vi "Create Parser.vi"(8 "error in (no error)":errorcluster, 10 "LVLIBP Path":path) -> (0 "error out":errorcluster, 3 "LVLIBP Parser out":refnum<class "LVLIBP Parser.lvclass">)   [LabVIEW 2020, in "LVLIBP CD XML Updater.lvlib" / "LVLIBP Parser.lvclass"]
uses:
  LVLIBP Parser.lvclass
  LVLIBP Parser.lvclass/LVLIBP Parser.ctl
  <vilib>/Utility/LVLibp/NI_PackedLibraryUtility.lvlib
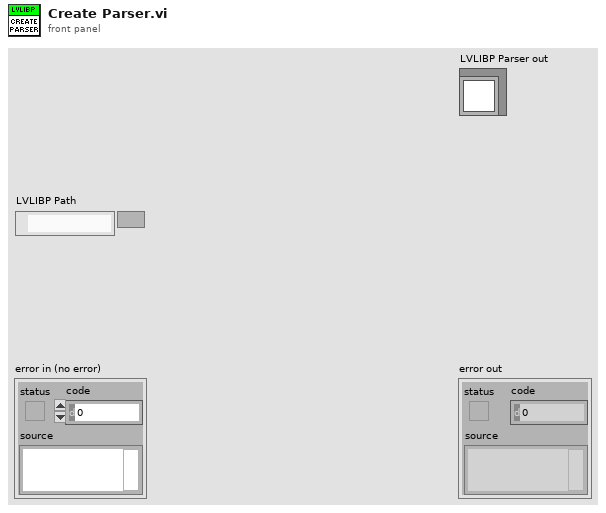
[diagram p1: front panel]
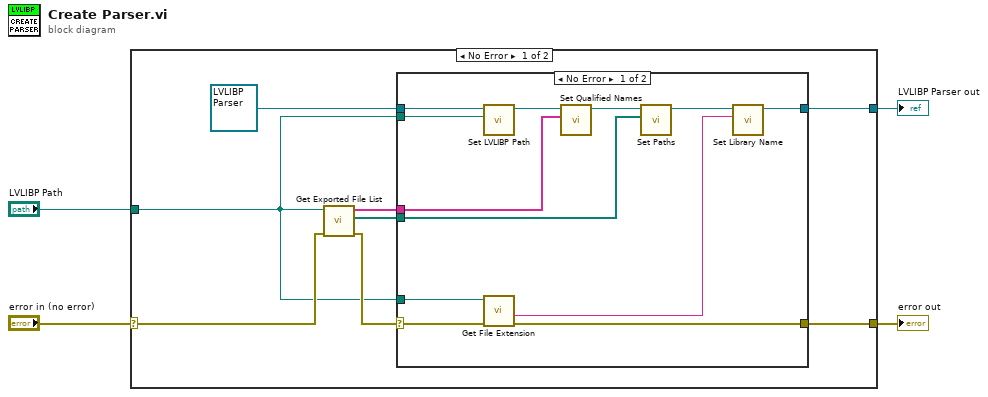
[diagram p0: block diagram]
diagram:
  n1 = case shown="No Error" "error in (no error)" {
    selector: "error in (no error)" -> [w10 w27]
    tunnel: [w8 w27] -> w3
    tunnel: "LVLIBP Path" -> [w5 _]
    tunnel: [w11 _] -> w1
    frame No Error {
      n2 = call <vilib>:"Get Exported File List.vi"("error in (no error)"=w10, "packed library path"=w5) -> ("error out"=w9:errorcluster, "paths"=w7:path[], "qualified names"=w6:string[])  [unwired: 7 in]
      n3 = case shown="No Error" w9 {
        selector: w9 -> [w20 w25]
        tunnel: refnum<class "LVLIBP Parser.lvclass"> refnum ("LVLIBP Parser out") -> [w24 w26]
        tunnel: w5 -> [w18 _]
        tunnel: [w14 w26] -> w11
        tunnel: [w19 w25] -> w8
        tunnel: w7 -> [w21 _]
        tunnel: w6 -> [w22 _]
        tunnel: w5 -> [w13 _]
        frame No Error {
          n4 = call "Set LVLIBP Path.vi"("LVLIBP Path"=w18, "LVLIBP Parser in"=w24) -> ("LVLIBP Parser out"=w16:refnum<class "LVLIBP Parser.lvclass">)  [unwired: 9 in]
          n5 = call <vilib>:"Get File Extension.vi"("error in (no error)"=w20, "file"=w13) -> ("error out"=w19:errorcluster, "filename without extension"=w17:string)  [unwired: 5 in, 3 out]
          n6 = call "Set Qualified Names.vi"("Qualified Names"=w22, "LVLIBP Parser in"=w16) -> ("LVLIBP Parser out"=w23:refnum<class "LVLIBP Parser.lvclass">)  [unwired: 9 in]
          n7 = call "Set Paths.vi"("Paths"=w21, "LVLIBP Parser in"=w23) -> ("LVLIBP Parser out"=w15:refnum<class "LVLIBP Parser.lvclass">)  [unwired: 9 in]
          n8 = call "Set Library Name.vi"("Library Name"=w17, "LVLIBP Parser in"=w15) -> ("LVLIBP Parser out"=w14:refnum<class "LVLIBP Parser.lvclass">)  [unwired: 9 in]
        }
        frame Error {
        }
      }
    }
    frame Error {
    }
  }
  "error out" <- w3
  "LVLIBP Parser out" <- w1
